vi "ClsSendCmds_String.vi"(8 "error in (no error)":errorcluster, 10 "Command In":string, 11 "Connection Out in":u32) -> (0 "error out":errorcluster, 2 "Command Response":string, 3 "Connection Out out":u32)   [LabVIEW 2015]
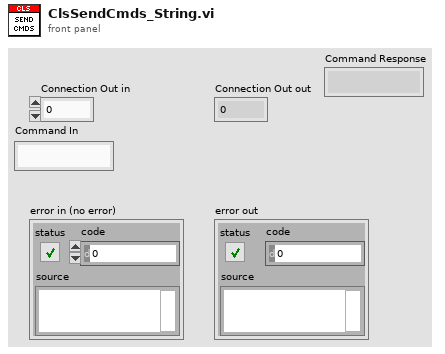
[diagram p1: front panel]
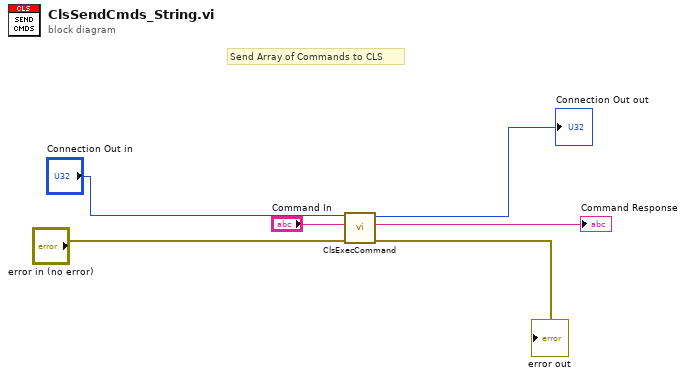
[diagram p0: block diagram]
diagram:
  # "Send Array of Commands to CLS"
  n1 = call "ClsExecCommand.vi"("error in (no error)"="error in (no error)", "Command In"="Command In", "Connection In"="Connection Out in") -> ("error out"=→"error out":errorcluster, "Command Response"=→"Command Response":string, "Connection Out"=→"Connection Out out":u32)  [unwired: 6 in]
